vi "FPGA Input Stimulus_5772.vi"(0 "sim I/O info in":T1, 9 "data from node input terminals":variant[](array[variant]), 11 "input from node terminal error in":errorcluster) -> (4 "sim I/O info out":T1, 10 "data to node output terminals":variant[](array[variant]), 15 "output to node terminal error out":errorcluster)   [LabVIEW 2011]
uses:
  <vilib>/FPGA/viExecutionOnDevComputer/simIO/customVI/Sim IO Info.ctl
  <vilib>/rvi/customViForEmulation/niLvFPGAUserSpecifiedEmulationVISupport.lvclass
  <vilib>/FPGA/viExecutionOnDevComputer/simIO/customVI/niFPGA Simulated IO.lvlib
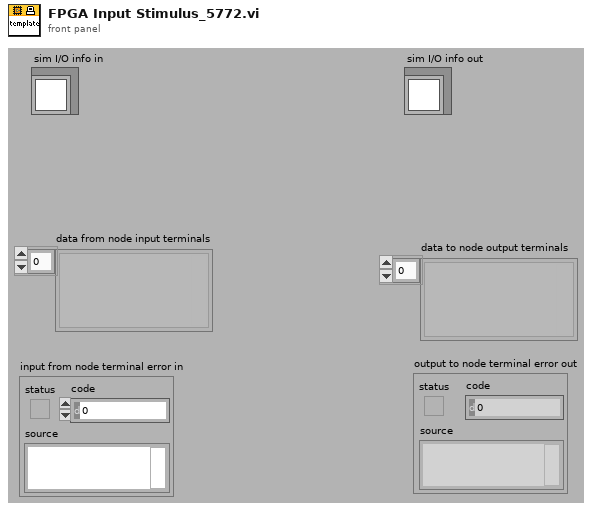
[diagram p1: front panel]
types:
  T1 = typedef "niFPGA Simulated IO.lvlib/Sim IO Info.ctl" = refnum<class "niLvFPGAUserSpecifiedEmulationVISupport.lvclass">
  T2 = typedef "niFPGA Simulated IO.lvlib/Execution Stage.ctl" = enum16{"Initializing", "Running", "Shutting Down"}
  T3 = typedef "niFPGA Simulated IO.lvlib/Node or Element Type.ctl" = enum16{"Read I/O", "Write I/O", "Method", "Read Property", "Write Property"}
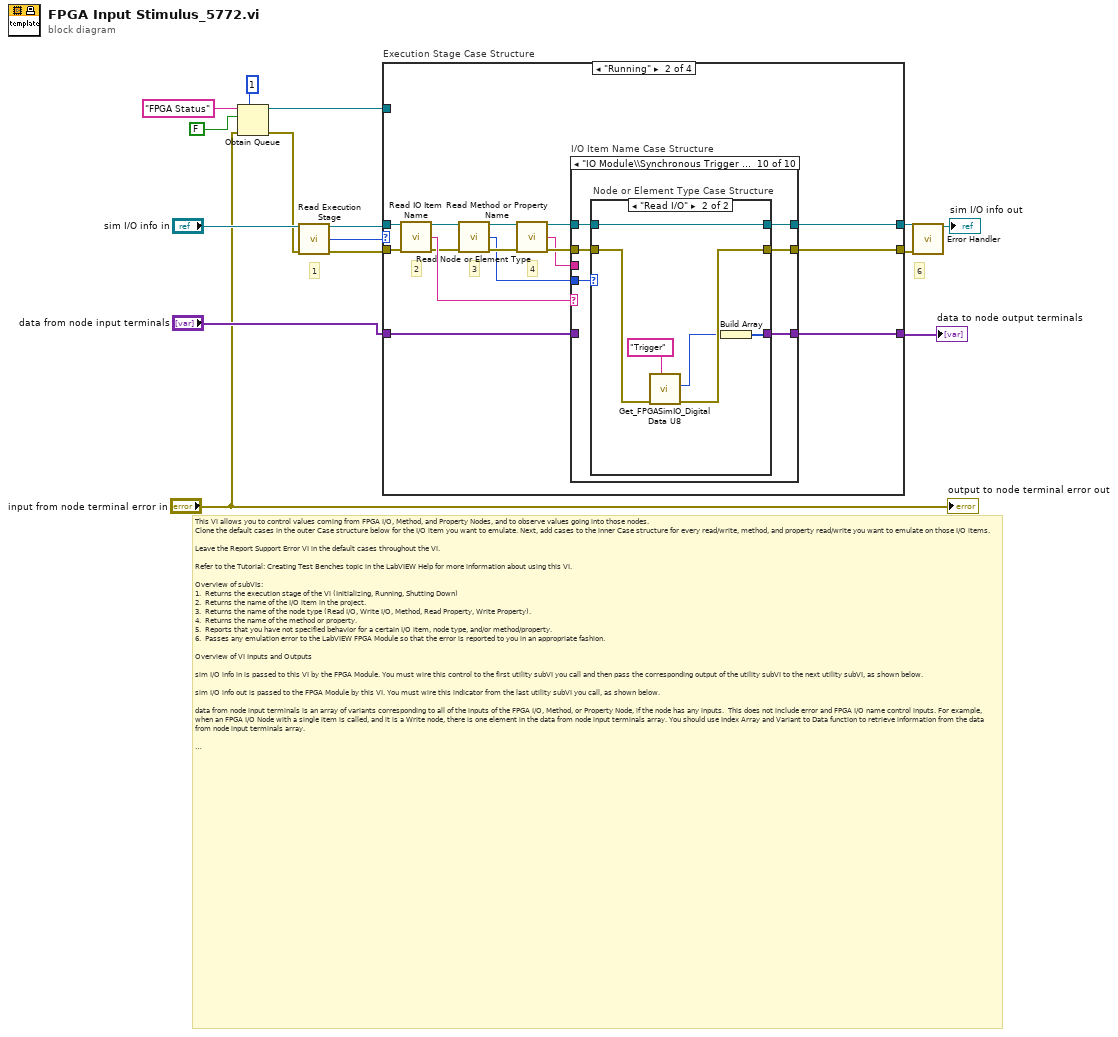
[diagram p0: block diagram]
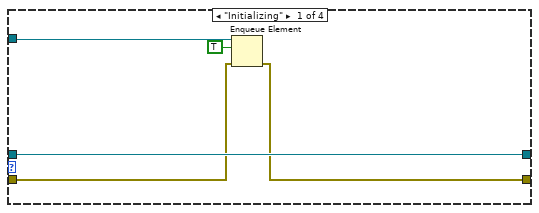
[diagram p2: hidden frame]
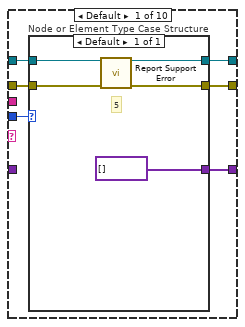
[diagram p3: hidden frame]
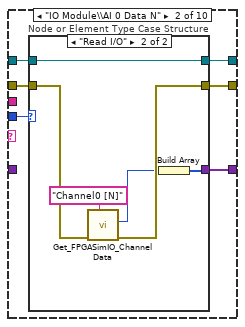
[diagram p4: hidden frame]
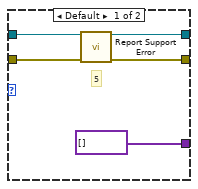
[diagram p5: hidden frame]
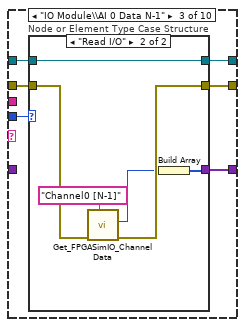
[diagram p6: hidden frame]
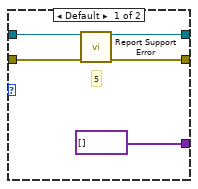
[diagram p7: hidden frame]
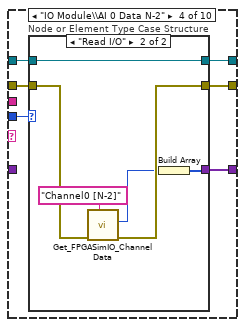
[diagram p8: hidden frame]
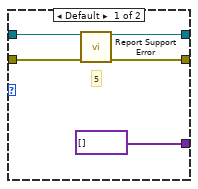
[diagram p9: hidden frame]
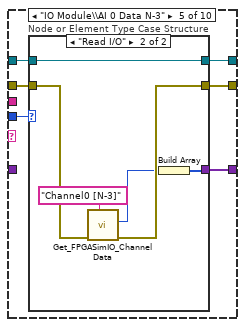
[diagram p10: hidden frame]
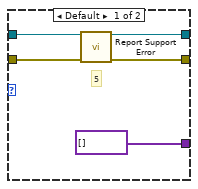
[diagram p11: hidden frame]
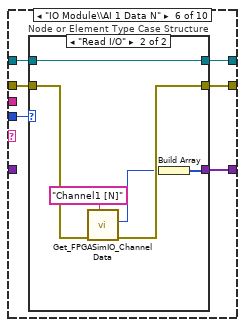
[diagram p12: hidden frame]
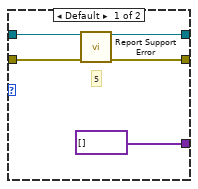
[diagram p13: hidden frame]
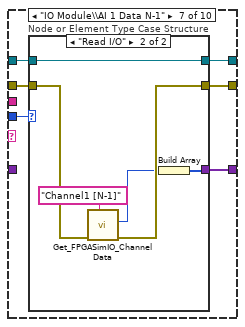
[diagram p14: hidden frame]
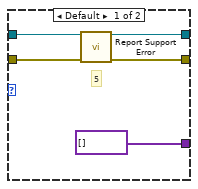
[diagram p15: hidden frame]
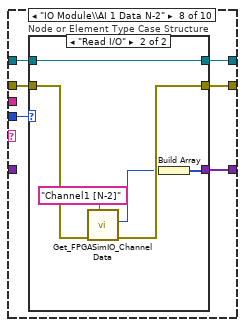
[diagram p16: hidden frame]
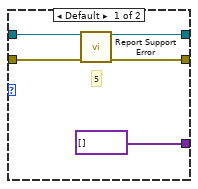
[diagram p17: hidden frame]
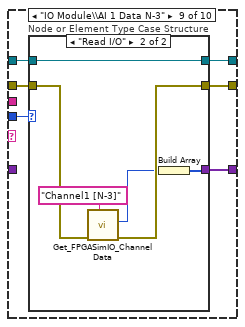
[diagram p18: hidden frame]
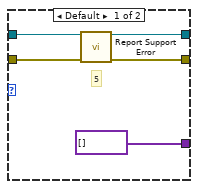
[diagram p19: hidden frame]
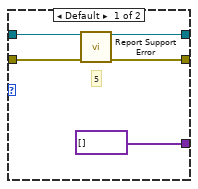
[diagram p20: hidden frame]
diagram:
  # "1"
  # "6"
  # "This VI allows you to control values coming from FPGA I/O, Method, and Property Nodes, and to observe values going into those nodes.\nClone the default cases in the outer Case structure below for the I/O item you want to emulate. Next, add cases to the inner Case structure for every read/write, method, and property read/write you want to emulate on those I/O items.  \n\nLeave the Report Support Error VI in the default cases throughout the VI.\n\nRefer to the Tutorial: Creating Test Benches topic in the LabVIEW Help for more information about using this VI.\n\nOverview of subVIs:\n1.  Returns the execution stage of the VI (Initializing, Running, Shutting Down)\n2.  Returns the name of the I/O item in the project.\n3.  Returns the name of the node type (Read I/O, Write I/O, Method, Read Property, Write Property).\n4.  Returns the name of the method or property.\n5.  Reports that you have not specified behavior for a certain I/O item, node type, and/or method/property.\n6.  Passes any emulation error to the LabVIEW FPGA Module so that the error is reported to you in an appropriate fashion.\n\nOverview of VI Inputs and Outputs\n\nsim I/O info in is passed to this VI by the FPGA Module. You must wire this control to the first utility subVI you call and then pass the corresponding output of the utility subVI to the next utility subVI, as shown below.\n\nsim I/O info out is passed to the FPGA Module by this VI. You must wire this indicator from the last utility subVI you call, as shown below.\n\ndata from node input terminals is an array of variants corresponding to all of the inputs of the FPGA I/O, Method, or Property Node, if the node has any inputs.  This does not include error and FPGA I/O name control inputs. For example, when an FPGA I/O Node with a single item is called, and it is a Write node, there is one element in the data from node input terminals array. You should use Index Array and Variant to Data function to retrieve information from the data from node input terminals array.\n\ndata to node output terminals is an array of variants corresponding to all the outputs of the FPGA I/O, Method, or Property Node, if the node has any outputs.  This does not include error and FPGA I/O name control outputs. For example, when an FPGA I/O node with a single item is called, and it is a Read node, there should be one element in the data to node output terminals array. You should use To Variant and Build Array functions to pass the information to the data to node output terminals array.\n\ninput from node terminal error in is the error that gets passed into the FPGA I/O, Method, or Property Node, if the node is configured so that the error input is shown. If the node is configured so that the error input is not shown, the value of this input corresponds to \"no error\" (status is false, error code is 0). \n\noutput to node terminal error out is the error that gets passed out of the FPGA I/O, Method, or Property Node, if the node is configured so that the error output is shown.  If the node is configured so that the error output is not shown, the value of this output is ignored."
  n1 = Obtain Queue(max queue size (-1, unlimited)=1, name (unnamed)="FPGA Status", element data type=FALSE, error in (no error)="input from node terminal error in") -> (queue out=w3:refnum<queue>, error out=w1:errorcluster)  [unwired: 1 in, 1 out]
  n2 = call <vilib>:"Read Execution Stage.vi"("sim I/O info in"="sim I/O info in", "error in (no error)"=w1) -> ("sim I/O info out"=w13:T1, "execution stage"=w12:T2, "error out"=w11:errorcluster)  [unwired: 11 out]
  n3 = case "Execution Stage Case Structure" shown="\"Running\"" w12 {
    tunnel: [_ w34 _ _] -> w7
    tunnel: [w17 w21 w200 w205] -> w9
    tunnel: [w20 w26 w203 w204] -> w8
    tunnel: w13 -> [w20 w24 w203 w204]
    tunnel: w11 -> [w18 w23 w201 w205]
    tunnel: "data from node input terminals" -> [_ w35 _ _]
    tunnel: w3 -> [w19 _ w202 _]
    frame "Initializing" {
      n4 = Enqueue Element(queue=w19, element=TRUE, error in (no error)=w18) -> (error out=w17:errorcluster)  [unwired: 1 in, 2 out]
    }
    frame "Running" {
      # "4"
      # "3"
      # "2"
      n5 = call <vilib>:"Read IO Item Name.vi"("sim I/O info in"=w24, "error in (no error)"=w23) -> ("sim I/O info out"=w25:T1, "I/O item name"=w33:string, "error out"=w32:errorcluster)  [unwired: 11 out]
      n6 = call <vilib>:"Read Node or Element Type.vi"("sim I/O info in"=w25, "error in (no error)"=w32) -> ("sim I/O info out"=w22:T1, "node or element type"=w30:T3, "error out"=w31:errorcluster)  [unwired: 11 out]
      n7 = call <vilib>:"Read Method or Property Name.vi"("sim I/O info in"=w22, "error in (no error)"=w31) -> ("sim I/O info out"=w28:T1, "method or property name"=w27:string, "error out"=w29:errorcluster)  [unwired: 11 out]
      n8 = case "I/O Item Name Case Structure" shown="\"IO Module\\\\Synchronous Trigger Input\"" w33 {
        tunnel: w35 -> [_ _ _ _ _ _ _ _ _ _]
        tunnel: [w37 w48 w65 w82 w99 w116 w133 w150 w167 w184] -> w34
        tunnel: w29 -> [w41 w52 w69 w86 w103 w120 w137 w154 w171 w188]
        tunnel: [w40 w51 w68 w85 w102 w119 w136 w153 w170 w187] -> w21
        tunnel: w28 -> [w39 w50 w67 w84 w101 w118 w135 w152 w169 w186]
        tunnel: [w38 w49 w66 w83 w100 w117 w134 w151 w168 w185] -> w26
        tunnel: w30 -> [w36 w47 w64 w81 w98 w115 w132 w149 w166 w183]
        tunnel: w27 -> [_ _ _ _ _ _ _ _ _ _]
        frame Default {
          n9 = case "Node or Element Type Case Structure" shown="Default" w36 {
            tunnel: w41 -> [w46]
            tunnel: [w45] -> w40
            tunnel: w39 -> [w44]
            tunnel: [w43] -> w38
            tunnel: [variant[] []] -> w37
            frame Default {
              # "5"
              n10 = call <vilib>:"Report Support Error.vi"("sim I/O info in"=w44, "error in (no error)"=w46) -> ("sim I/O info out"=w43:T1, "error out"=w45:errorcluster)  [unwired: 12 out]
            }
          }
        }
        frame "IO Module\\AI 0 Data N" {
          n11 = case "Node or Element Type Case Structure" shown="\"Read I/O\"" w47 {
            tunnel: w52 -> [w57 w61]
            tunnel: [w56 w60] -> w51
            tunnel: w50 -> [w55 w63]
            tunnel: [w54 w63] -> w49
            tunnel: [variant[] [] w62] -> w48
            frame Default {
              # "5"
              n12 = call <vilib>:"Report Support Error.vi"("sim I/O info in"=w55, "error in (no error)"=w57) -> ("sim I/O info out"=w54:T1, "error out"=w56:errorcluster)  [unwired: 12 out]
            }
            frame "Read I/O" {
              n13 = call <userlib>:"Get_FPGASimIO_Channel Data.vi"("Channel Name"="Channel0 [N]", "Error In"=w61) -> ("Error Out"=w60:errorcluster, "Data"=w59:i16)  [unwired: 8 in]
              n14 = Build Array(w59) -> (w62:i16[])
            }
          }
        }
        frame "IO Module\\AI 0 Data N-1" {
          n15 = case "Node or Element Type Case Structure" shown="\"Read I/O\"" w64 {
            tunnel: w69 -> [w74 w78]
            tunnel: [w73 w77] -> w68
            tunnel: w67 -> [w72 w80]
            tunnel: [w71 w80] -> w66
            tunnel: [variant[] [] w79] -> w65
            frame Default {
              # "5"
              n16 = call <vilib>:"Report Support Error.vi"("sim I/O info in"=w72, "error in (no error)"=w74) -> ("sim I/O info out"=w71:T1, "error out"=w73:errorcluster)  [unwired: 12 out]
            }
            frame "Read I/O" {
              n17 = call <userlib>:"Get_FPGASimIO_Channel Data.vi"("Channel Name"="Channel0 [N-1]", "Error In"=w78) -> ("Error Out"=w77:errorcluster, "Data"=w76:i16)  [unwired: 8 in]
              n18 = Build Array(w76) -> (w79:i16[])
            }
          }
        }
        frame "IO Module\\AI 0 Data N-2" {
          n19 = case "Node or Element Type Case Structure" shown="\"Read I/O\"" w81 {
            tunnel: w86 -> [w91 w95]
            tunnel: [w90 w94] -> w85
            tunnel: w84 -> [w89 w97]
            tunnel: [w88 w97] -> w83
            tunnel: [variant[] [] w96] -> w82
            frame Default {
              # "5"
              n20 = call <vilib>:"Report Support Error.vi"("sim I/O info in"=w89, "error in (no error)"=w91) -> ("sim I/O info out"=w88:T1, "error out"=w90:errorcluster)  [unwired: 12 out]
            }
            frame "Read I/O" {
              n21 = call <userlib>:"Get_FPGASimIO_Channel Data.vi"("Channel Name"="Channel0 [N-2]", "Error In"=w95) -> ("Error Out"=w94:errorcluster, "Data"=w93:i16)  [unwired: 8 in]
              n22 = Build Array(w93) -> (w96:i16[])
            }
          }
        }
        frame "IO Module\\AI 0 Data N-3" {
          n23 = case "Node or Element Type Case Structure" shown="\"Read I/O\"" w98 {
            tunnel: w103 -> [w108 w112]
            tunnel: [w107 w111] -> w102
            tunnel: w101 -> [w106 w114]
            tunnel: [w105 w114] -> w100
            tunnel: [variant[] [] w113] -> w99
            frame Default {
              # "5"
              n24 = call <vilib>:"Report Support Error.vi"("sim I/O info in"=w106, "error in (no error)"=w108) -> ("sim I/O info out"=w105:T1, "error out"=w107:errorcluster)  [unwired: 12 out]
            }
            frame "Read I/O" {
              n25 = call <userlib>:"Get_FPGASimIO_Channel Data.vi"("Channel Name"="Channel0 [N-3]", "Error In"=w112) -> ("Error Out"=w111:errorcluster, "Data"=w110:i16)  [unwired: 8 in]
              n26 = Build Array(w110) -> (w113:i16[])
            }
          }
        }
        frame "IO Module\\AI 1 Data N" {
          n27 = case "Node or Element Type Case Structure" shown="\"Read I/O\"" w115 {
            tunnel: w120 -> [w125 w129]
            tunnel: [w124 w128] -> w119
            tunnel: w118 -> [w123 w131]
            tunnel: [w122 w131] -> w117
            tunnel: [variant[] [] w130] -> w116
            frame Default {
              # "5"
              n28 = call <vilib>:"Report Support Error.vi"("sim I/O info in"=w123, "error in (no error)"=w125) -> ("sim I/O info out"=w122:T1, "error out"=w124:errorcluster)  [unwired: 12 out]
            }
            frame "Read I/O" {
              n29 = call <userlib>:"Get_FPGASimIO_Channel Data.vi"("Channel Name"="Channel1 [N]", "Error In"=w129) -> ("Error Out"=w128:errorcluster, "Data"=w127:i16)  [unwired: 8 in]
              n30 = Build Array(w127) -> (w130:i16[])
            }
          }
        }
        frame "IO Module\\AI 1 Data N-1" {
          n31 = case "Node or Element Type Case Structure" shown="\"Read I/O\"" w132 {
            tunnel: w137 -> [w142 w146]
            tunnel: [w141 w145] -> w136
            tunnel: w135 -> [w140 w148]
            tunnel: [w139 w148] -> w134
            tunnel: [variant[] [] w147] -> w133
            frame Default {
              # "5"
              n32 = call <vilib>:"Report Support Error.vi"("sim I/O info in"=w140, "error in (no error)"=w142) -> ("sim I/O info out"=w139:T1, "error out"=w141:errorcluster)  [unwired: 12 out]
            }
            frame "Read I/O" {
              n33 = call <userlib>:"Get_FPGASimIO_Channel Data.vi"("Channel Name"="Channel1 [N-1]", "Error In"=w146) -> ("Error Out"=w145:errorcluster, "Data"=w144:i16)  [unwired: 8 in]
              n34 = Build Array(w144) -> (w147:i16[])
            }
          }
        }
        frame "IO Module\\AI 1 Data N-2" {
          n35 = case "Node or Element Type Case Structure" shown="\"Read I/O\"" w149 {
            tunnel: w154 -> [w159 w163]
            tunnel: [w158 w162] -> w153
            tunnel: w152 -> [w157 w165]
            tunnel: [w156 w165] -> w151
            tunnel: [variant[] [] w164] -> w150
            frame Default {
              # "5"
              n36 = call <vilib>:"Report Support Error.vi"("sim I/O info in"=w157, "error in (no error)"=w159) -> ("sim I/O info out"=w156:T1, "error out"=w158:errorcluster)  [unwired: 12 out]
            }
            frame "Read I/O" {
              n37 = call <userlib>:"Get_FPGASimIO_Channel Data.vi"("Channel Name"="Channel1 [N-2]", "Error In"=w163) -> ("Error Out"=w162:errorcluster, "Data"=w161:i16)  [unwired: 8 in]
              n38 = Build Array(w161) -> (w164:i16[])
            }
          }
        }
        frame "IO Module\\AI 1 Data N-3" {
          n39 = case "Node or Element Type Case Structure" shown="\"Read I/O\"" w166 {
            tunnel: w171 -> [w176 w180]
            tunnel: [w175 w179] -> w170
            tunnel: w169 -> [w174 w182]
            tunnel: [w173 w182] -> w168
            tunnel: [variant[] [] w181] -> w167
            frame Default {
              # "5"
              n40 = call <vilib>:"Report Support Error.vi"("sim I/O info in"=w174, "error in (no error)"=w176) -> ("sim I/O info out"=w173:T1, "error out"=w175:errorcluster)  [unwired: 12 out]
            }
            frame "Read I/O" {
              n41 = call <userlib>:"Get_FPGASimIO_Channel Data.vi"("Channel Name"="Channel1 [N-3]", "Error In"=w180) -> ("Error Out"=w179:errorcluster, "Data"=w178:i16)  [unwired: 8 in]
              n42 = Build Array(w178) -> (w181:i16[])
            }
          }
        }
        frame "IO Module\\Synchronous Trigger Input" {
          n43 = case "Node or Element Type Case Structure" shown="\"Read I/O\"" w183 {
            tunnel: w188 -> [w193 w197]
            tunnel: [w192 w196] -> w187
            tunnel: w186 -> [w191 w199]
            tunnel: [w190 w199] -> w185
            tunnel: [variant[] [] w198] -> w184
            frame Default {
              # "5"
              n44 = call <vilib>:"Report Support Error.vi"("sim I/O info in"=w191, "error in (no error)"=w193) -> ("sim I/O info out"=w190:T1, "error out"=w192:errorcluster)  [unwired: 12 out]
            }
            frame "Read I/O" {
              n45 = call <userlib>:"Get_FPGASimIO_Digital Data U8.vi"("Channel Name"="Trigger", "Error In"=w197) -> ("Error Out"=w196:errorcluster, "Data"=w195:u8)  [unwired: 8 in]
              n46 = Build Array(w195) -> (w198:u8[])
            }
          }
        }
      }
    }
    frame "Shutting Down" {
      n47 = Flush Queue(queue=w202, error in (no error)=w201) -> (error out=w200:errorcluster)  [unwired: 2 out]
    }
    frame Default {
    }
  }
  "data to node output terminals" <- w7
  n48 = call <vilib>:"Error Handler.vi"("sim I/O info in"=w8, "error in"=w9) -> ("sim I/O info out"=→"sim I/O info out":T1)  [unwired: 13 out]
  "output to node terminal error out" <- "input from node terminal error in"
